vi "SQL_复制已有表至指定表.vi"(8 "error in (no error)":errorcluster caption="错误输入（无错误）", 10 "已有表名":string="d7", 11 "新表名":string="test") -> (0 "error out":errorcluster caption="错误输出", 3 "SQL_复制已有表至指定表":string)   [LabVIEW 2014]
doc: "该模板用于创建子VI。"
panel:
  # "varchar括号中的数值最大255"
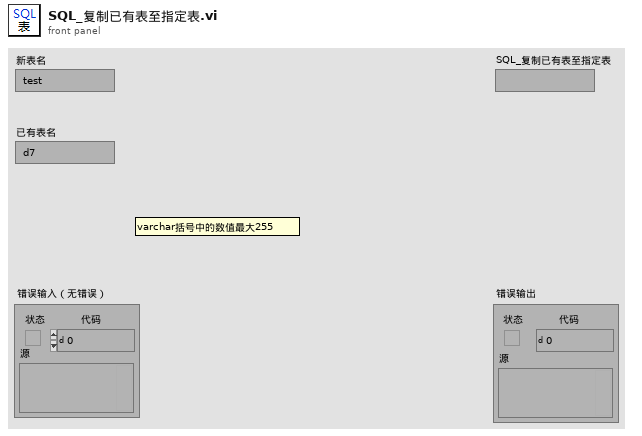
[diagram p1: front panel]
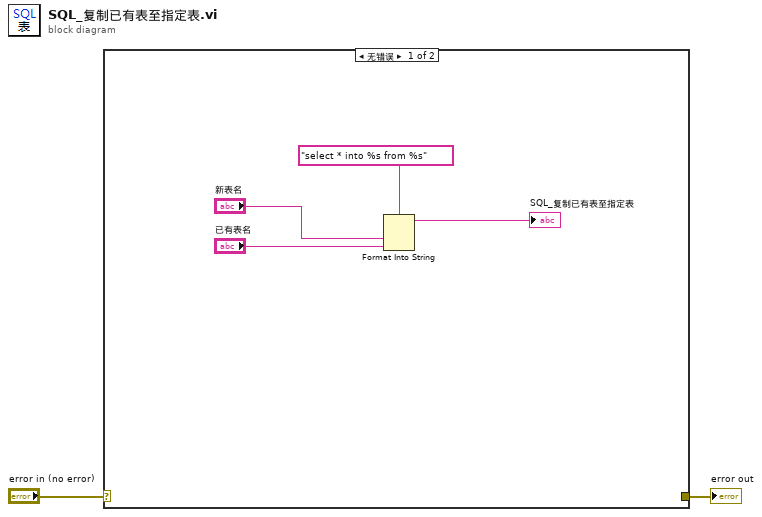
[diagram p0: block diagram]
diagram:
  n1 = case shown="无错误" "error in (no error)" {
    selector: "error in (no error)" -> [_ w7]
    tunnel: [_ w7] -> w1
    frame No Error {
      n2 = Format Into String(format string="select * into %s from %s", "新表名", "已有表名") -> (resulting string=→"SQL_复制已有表至指定表":string)  [unwired: 2 in, 1 out]
    }
    frame Error {
    }
  }
  "error out" <- w1
